vi "Init Waveform DVRs.vi"(8 "error in (no error)":errorcluster) -> (0 "error out":errorcluster, 3 "Waveform":T1)   [LabVIEW 2021, in "BT.lvlib" / "bt_Blackboard.lvclass"]
uses:
  Status Type.ctl
  bt_Blackboard.lvclass
  bt_Blackboard.lvclass/bt_Blackboard.ctl
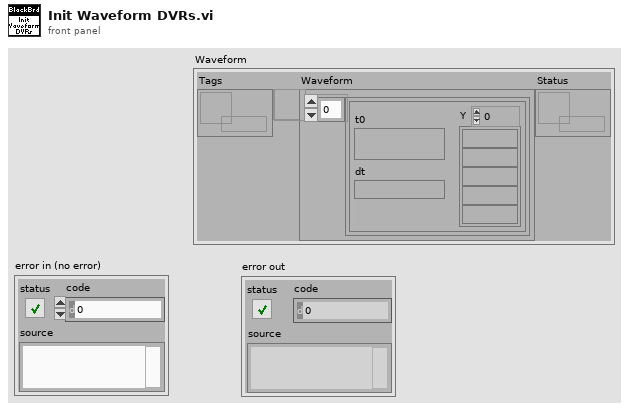
[diagram p1: front panel]
types:
  T1 = cluster{"Tags":refnum<data-value>, "Waveform":refnum<data-value>, "Status":refnum<data-value>}
  T2 = typedef "BT.lvlib/bt_Blackboard.lvclass/Status Type.ctl" = cluster{"Read?":bool, "Write?":bool}
  T3 = cluster{"Tags":refnum<data-value>, "Waveform ":refnum<data-value>, "Status":refnum<data-value>}
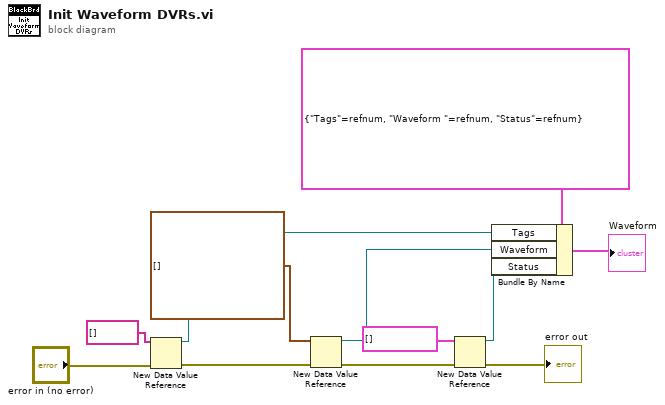
[diagram p0: block diagram]
diagram:
  n1 = New Data Value Reference(data value=string[] [], error in="error in (no error)") -> (data value reference=w8:refnum<data-value>, error out=w10:errorcluster)
  n2 = New Data Value Reference(data value=waveform(dbl)[] [], error in=w10) -> (data value reference=w7:refnum<data-value>, error out=w5:errorcluster)
  n3 = New Data Value Reference(data value=T2[] [] ("Array"), error in=w5) -> (data value reference=w4:refnum<data-value>, error out=→"error out":errorcluster)
  n4 = Bundle By Name(cluster=T3 {"Tags"=refnum, "Waveform "=refnum, "Status"=refnum} ("Boolean"), "Tags"=w8, "Waveform"=w7, "Status"=w4) -> (→"Waveform":T3)
